vi "startStopPulsator.vi"(8 "comms":T1, 9 "message scheduler":refnum<class "message scheduler.lvclass">, 10 "start?":variant, 11 "Queues":T2) -> (0 "comms out":T1)   [LabVIEW 2018]
uses:
  type defs/comms loop data.ctl
  ICL-LabVIEW_General/Incident logger/Incident logger.lvclass
  <vilib>/Modbus/master/Modbus Master.lvclass
  type defs/Queues.ctl
  ICL-LabVIEW_General/Message Scheduler/message scheduler.lvclass
  ICL-LabVIEW_General/Message Scheduler/generic message queue/standard message queue/standard message.lvclass
  D:/Chris/oneDrive/OneDrive - Imperial College London/LabVIEW/Chris VIs/Message Scheduler/generic message queue/generic message.lvclass
  <vilib>/Utility/error.llb/Error Cluster From Error Code.vi
  ICL-LabVIEW_General/Pulser Controller/AKD MODBUS commands/stop drive.vi
  ICL-LabVIEW_General/Pulser Controller/AKD MODBUS commands/start drive.vi
  <vilib>/ErrorRing/Error Ring.xnode
  ICL-LabVIEW_General/Pulser Controller/Pulser controller commands library.lvlib
  ICL-LabVIEW_General/Message Scheduler/scheduled message/scheduled message.lvclass
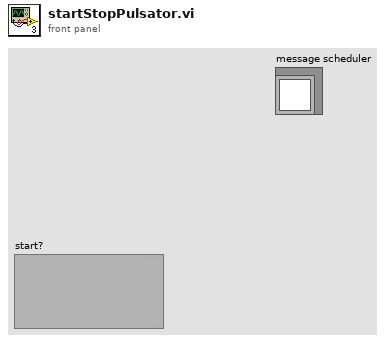
[diagram p1: front panel]
types:
  T1 = typedef "comms loop data.ctl" = cluster{"params":cluster{"commandStream":cluster{"reader name":string, "writer name":string, "stream buffer size":i32}, "errorStream":cluster{"reader name":string, "writer name":string, "stream buffer size":i32}, "RT IP address":string, "pulserControllerIP":string}, "vars":cluster{"commandStream":refnum<k21>, "Incident logger":refnum<class "Incident logger.lvclass">, "check error scheduled message":u32, "errorStream":refnum<k21>, "watchdogScheduleID":u32, "pulsator":cluster{"pulser connection":refnum<class "Modbus Master.lvclass">, "pulserConnected":bool, "pulsatorScheduleID":u32, "pulserRunning":bool}}}
  T2 = typedef "Queues.ctl" = cluster{"messageHandler":refnum<queue>, "comms":refnum<queue>, "dataStream":refnum<queue>, "dataProcessor":refnum<queue>, "fileIO":refnum<queue>, "userInterface":refnum<queue>, "errors":refnum<queue>, "customCompressor":refnum<queue>}
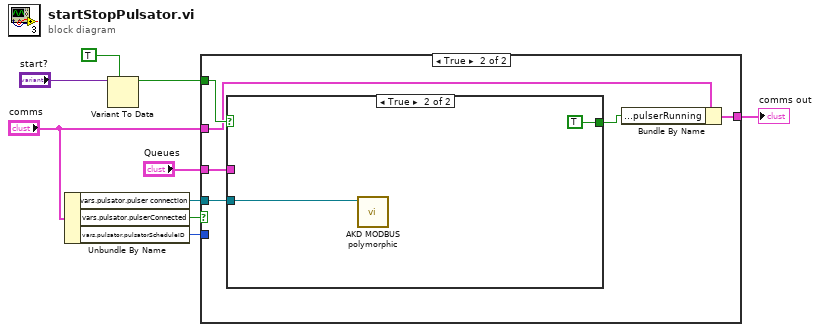
[diagram p0: block diagram]
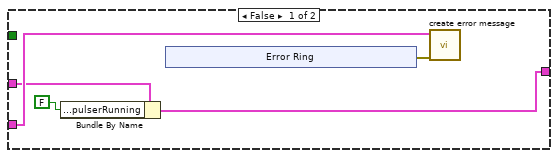
[diagram p2: hidden frame]
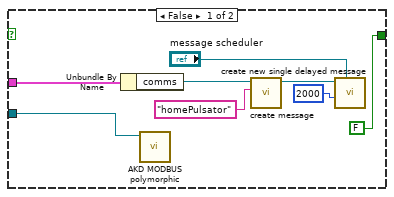
[diagram p3: hidden frame]
diagram:
  n1 = Unbundle By Name("comms") -> ("vars.pulsator.pulser connection"=w7:refnum<class "Modbus Master.lvclass">, "vars.pulsator.pulserConnected"=w9:bool, "vars.pulsator.pulsatorScheduleID"=w8:u32)
  n2 = Variant To Data(type=TRUE, Variant="start?") -> (data=w4:bool)  [unwired: 1 in, 1 out]
  n3 = case shown="True" w9 {
    tunnel: w8 -> [_ _]
    tunnel: w7 -> [_ w25]
    tunnel: "Queues" -> [w14 w23]
    tunnel: w4 -> [_ w24]
    tunnel: [w11 w21] -> w2
    tunnel: "comms" -> [w12 w22]
    frame False {
      n4 = Bundle By Name(cluster=w12, "vars.pulsator.pulserRunning"=FALSE) -> (w11:T1)
      n5 = xnode "Error Ring"() -> ("error out"=w13:errorcluster)
      n6 = call "create error message.vi"("error in (no error)"=w13, "queues"=w14) -> ()  [unwired: 10 in]
    }
    frame True {
      n7 = case shown="True" w24 {
        tunnel: w25 -> [w33 w35]
        tunnel: w23 -> [w32 _]
        tunnel: [FALSE TRUE] -> w20
        frame False {
          n8 = Unbundle By Name(w32) -> ("comms"=w31:refnum<queue>)
          n9 = call-poly "AKD MODBUS polymorphic.vi"("Modbus Master in"=w33) -> ()  [unwired: 10 in, 1 out]
          n10 = call "create message.vi"("message"="homePulsator", "queue ref"=w31) -> ("standard message out"=w29:refnum<class "standard message.lvclass">)  [unwired: 8 in, 1 out]
          n11 = call "create new single delayed message.vi"("message scheduler"="message scheduler", "ms delay"=u32 2000, "generic message queue.lvclass"=w29) -> ()  [unwired: 8 in, 1 out]
        }
        frame True {
          n12 = call-poly "AKD MODBUS polymorphic.vi"("Modbus Master in"=w35) -> ()  [unwired: 10 in, 1 out]
        }
      }
      n13 = Bundle By Name(cluster=w22, "vars.pulsator.pulserRunning"=w20) -> (w21:T1)
    }
  }
  "comms out" <- w2
